vi "Wave1D_Check Input_BC.vi"(8 "error in (no error)":errorcluster, 10 "Domain":T2={"t"={"initial t"=0.0, "final t"=1.0, "# of t-points"=11}, "x"={"start x"=0.0, "end x"=1.0, "# of x-points"=11}}, 11 "Boundary Condition":cluster{"type":T1, "Value":dbl[]}[](array[cluster]) {"type" items=["Dirichlet", "Neumann"]}) -> (0 "error out":errorcluster)   [LabVIEW 2020, in "NI_PDE.lvlib"]
uses:
  <vilib>/gmath/NI_PDE.lvlib
  <vilib>/gmath/pde.llb/Common/PDE_BC Type.ctl
  <vilib>/gmath/pde.llb/Common/PDE_Error.ctl
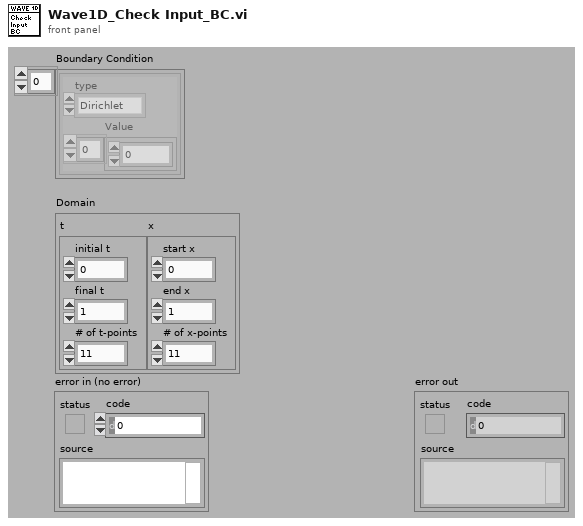
[diagram p1: front panel]
types:
  T1 = typedef "NI_PDE.lvlib/PDE_BC Type.ctl" = i32
  T2 = cluster{"t":cluster{"initial t":dbl, "final t":dbl, "# of t-points":i32}, "x":cluster{"start x":dbl, "end x":dbl, "# of x-points":i32}}
  T3 = typedef "NI_PDE.lvlib/PDE_Error.ctl" = enum16{"No Error", "k is zero", "End point <= start point", "# of time steps < 2", "# of spatial points < 3", "# of grid < 1 for FEM", "# of boundary < 3 for FEM", "Incompatible RHS size", "Incompatible BC size", "Incompatible IC size", "PDE class conflict", "RHS class conflict", "Domain class conflict", "BC class conflict", "IC class conflict"}
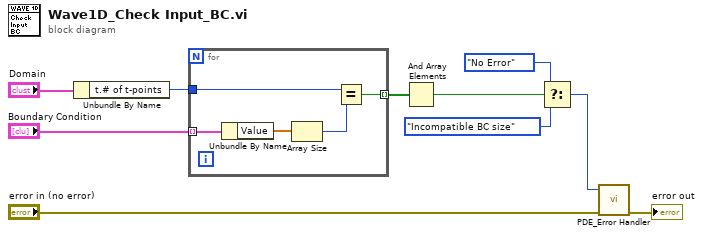
[diagram p0: block diagram]
diagram:
  n1 = Unbundle By Name("Domain") -> ("t.# of t-points"=w6:i32)
  n2 = for {
    tunnel: "Boundary Condition" -> [w15] mode=indexing
    tunnel: w6 -> [w13]
    tunnel: [w11] -> w5 mode=indexing
    n3 = Unbundle By Name(w15) -> ("Value"=w14:dbl[])
    n4 = Array Size(array=w14) -> (size(s)=w12:i32)
    n5 = Equal?(x=w13, y=w12) -> (x = y?=w11:bool)
  }
  n6 = And Array Elements(Boolean array=w5) -> (logical AND=w4:bool)
  n7 = Select(t=PDE_Error."No Error" ("Error"), s=w4, f=PDE_Error."Incompatible BC size" ("Error")) -> (s? t:f=w1:T3)
  n8 = call <vilib>:"PDE_Error Handler.vi"("error in (no error)"="error in (no error)", "PDE error"=w1) -> ("error out"=→"error out":errorcluster)  [unwired: 9 out]
